vi "4.5.vi"() -> ()   [LabVIEW 2017]
panel:
  out "循坏执行的次数":dbl
  in  "指定值":dbl
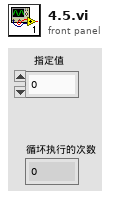
[diagram p1: front panel]
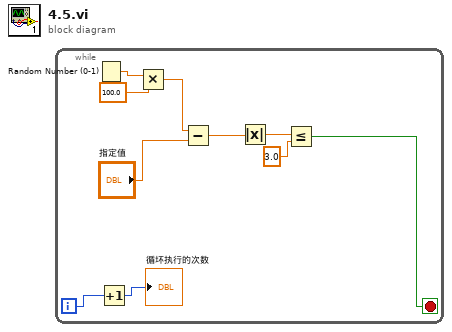
[diagram p0: block diagram]
diagram:
  n1 = while {
    i -> [w2]
    stop <- w3 stop-if-true
    n2 = Random Number (0-1)() -> (number: 0 to 1=w10:dbl)
    n3 = Increment(x=w2) -> (x+1=→"循坏执行的次数":i32)
    n4 = Multiply(x=w10, y=100.0) -> (x*y=w8:dbl)
    n5 = Subtract(x=w8, y="指定值") -> (x-y=w6:dbl)
    n6 = Absolute Value(x=w6) -> (abs(x)=w5:dbl)
    n7 = Less Or Equal?(x=w5, y=3.0) -> (x <= y?=w3:bool)
  }
